vi "mpps_data_to_plot.vi"(11 "Data Array":dbl[][](array[numeric])) -> (3 "JV Curve":cluster{"Y":dbl[], "Y":dbl[]}[](graph))   [LabVIEW 2016]
panel:
  in  "Tab Control 4":enum32{"Page 1"}(tab)
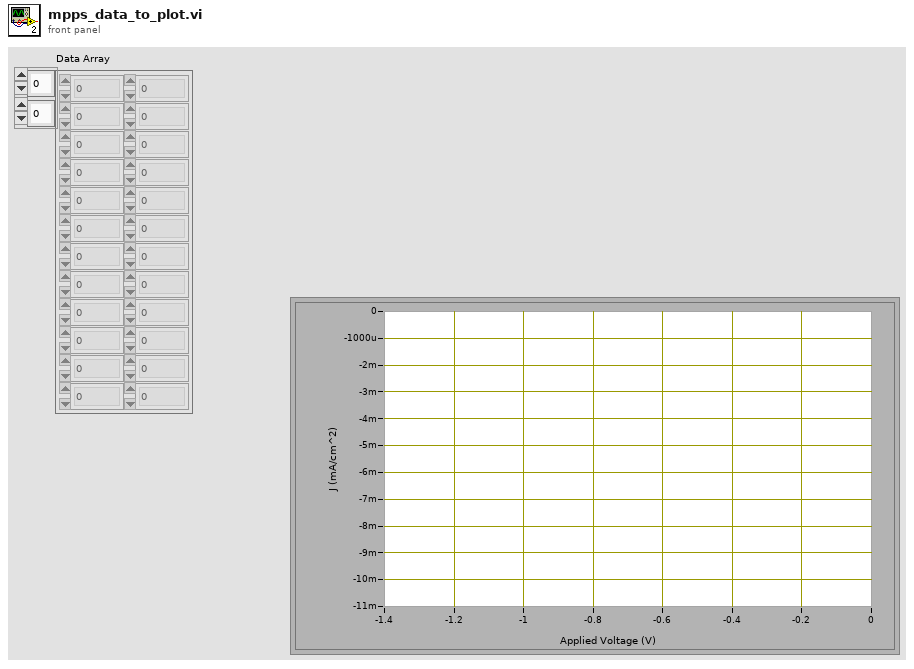
[diagram p1: front panel]
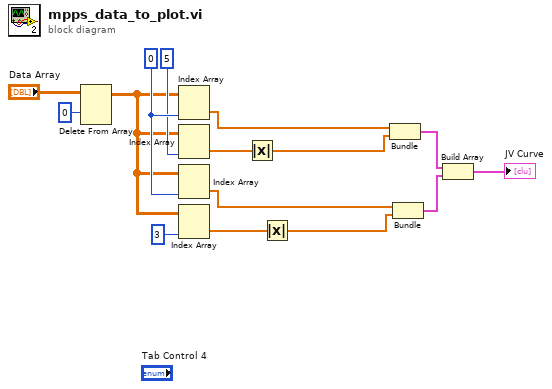
[diagram p0: block diagram]
diagram:
  w10 = 0
  n1 = Delete From Array(array="Data Array", index (row)=0) -> (array with subset deleted=w2:dbl[][])  [unwired: 2 in, 1 out]
  n2 = Index Array(array=w2, index (col)=w10) -> (element=w15:dbl[])  [unwired: 1 in]
  n3 = Index Array(array=w2, index (col)=5) -> (element=w5:dbl[])  [unwired: 1 in]
  n4 = Index Array(array=w2, index (col)=w10) -> (element=w14:dbl[])  [unwired: 1 in]
  n5 = Index Array(array=w2, index (col)=3 ("disabled index (col)")) -> (element=w7:dbl[])  [unwired: 1 in]
  n6 = Absolute Value(x=w5) -> (abs(x)=w4:dbl[])
  n7 = Absolute Value(x=w7) -> (abs(x)=w6:dbl[])
  n8 = Bundle("Data Array"=w15, w4) -> (w12:cluster{"Data Array":dbl[], dbl[]})  [unwired: 1 in]
  n9 = Bundle("Data Array"=w14, w6) -> (w13:cluster{"Data Array":dbl[], dbl[]})  [unwired: 1 in]
  n10 = Build Array(w12, w13) -> (→"JV Curve":cluster{"Data Array":dbl[], dbl[]}[])
